vi "步响应谷值.vi"(0 "行程 in":dbl[](array[numeric]), 2 "X_start":dbl, 3 "step_valley":dbl, 4 "（要求）连续大于0的次数":dbl=10.0) -> (5 "行程 out":dbl[](array[numeric]), 6 "X_value":dbl, 7 "X_value_next":dbl)   [LabVIEW 2013]
panel:
  out "连续大于0的次数":dbl=10.0
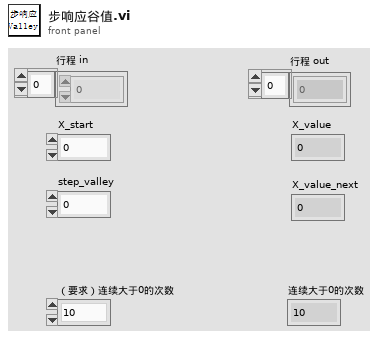
[diagram p1: front panel]
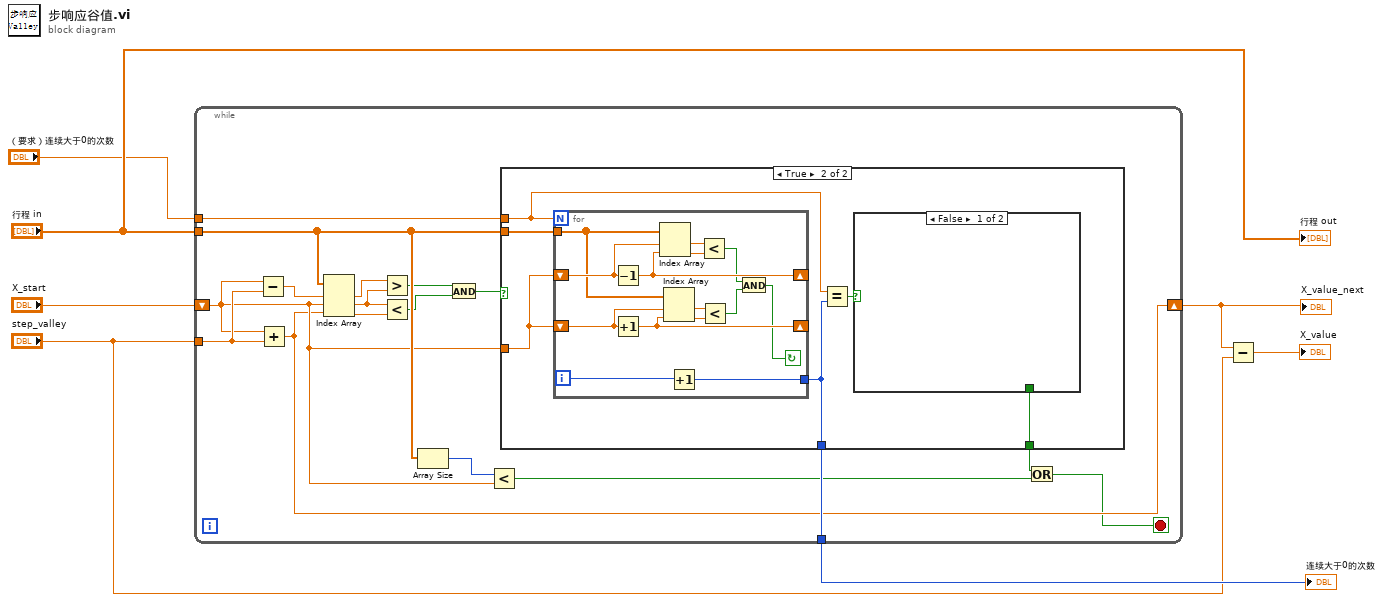
[diagram p0: block diagram]
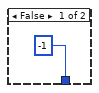
[diagram p2: hidden frame]
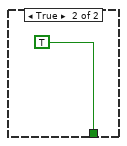
[diagram p3: hidden frame]
diagram:
  n1 = while {
    tunnel: "行程 in" -> [w19]
    shift-right: [w16] -> w1
    shift-left: "X_start" -> [w17]
    tunnel: "step_valley" -> [w24]
    tunnel: "（要求）连续大于0的次数" -> [w21]
    tunnel: [w20] -> w4
    stop <- w15 stop-if-true
    n2 = Subtract(x=w17, y=w24) -> (x-y=w23:dbl)
    n3 = Add(x=w17, y=w24) -> (x+y=w16:dbl)
    n4 = Index Array(array=w19, index #1=w23, index #2=w17, index #3=w16) -> (element #1=w12:dbl, element #2=w10:dbl, element #3=w8:dbl)
    n5 = Greater?(x=w12, y=w10) -> (0:w11:bool)
    n6 = Less?(x=w10, y=w8) -> (x < y?=w9:bool)
    n7 = Array Size(array=w19) -> (size(s)=w18:i32)
    n8 = And(x=w11, y=w9) -> (x .and. y?=w22:bool)
    n9 = Less?(x=w18, y=w17) -> (x < y?=w13:bool)
    n10 = case shown="True" w22 {
      tunnel: w17 -> [_ w29]
      tunnel: w21 -> [_ w30]
      tunnel: w19 -> [_ w31]
      tunnel: [-1 w28] -> w20
      tunnel: [_ w26] -> w14
      frame False {
      }
      frame True {
        n11 = for {
          N: w30 -> [_]
          shift-right: [w44] -> _
          shift-left: w29 -> [w43]
          shift-right: [w46] -> _
          shift-left: w29 -> [w45]
          tunnel: w31 -> [w38]
          tunnel: [w33] -> w28
          i -> [w34]
          stop <- w35 continue-if-true
          n12 = Decrement(x=w45) -> (x-1=w46:dbl)
          n13 = Increment(x=w43) -> (x+1=w44:dbl)
          n14 = Index Array(array=w38, index #1=w45, index #2=w46) -> (element #1=w42:dbl, element #2=w41:dbl)
          n15 = Index Array(array=w38, index #1=w43, index #2=w44) -> (element #1=w40:dbl, element #2=w39:dbl)
          n16 = Increment(x=w34) -> (x+1=w33:i32)
          n17 = Less?(x=w42, y=w41) -> (x < y?=w36:bool)
          n18 = Less?(x=w40, y=w39) -> (x < y?=w37:bool)
          n19 = And(x=w36, y=w37) -> (x .and. y?=w35:bool)
        }
        n20 = Equal?(x=w30, y=w28) -> (x = y?=w27:bool)
        n21 = case shown="False" w27 {
          tunnel: [_ TRUE] -> w26
          frame False {
          }
          frame True {
          }
        }
      }
    }
    n22 = Or(x=w14, y=w13) -> (x .or. y?=w15:bool)
  }
  "连续大于0的次数" <- w4
  "X_value_next" <- w1
  n23 = Subtract(x=w1, y="step_valley") -> (x-y=→"X_value":dbl)
  "行程 out" <- "行程 in"
